vi "client.vi"() -> ()   [LabVIEW 2019]
uses:
  Generated_client/RPC Messages/Greeter_req.ctl
  Generated_client/RPC Messages/Greeter_req_req_oneof/Greeter_req_req_oneof.lvclass
  Generated_client/RPC Messages/Greeter_req_req_oneof/Greeter_req_req_oneof.lvclass/Greeter_req_req_oneof.ctl
  Generated_client/RPC Messages/Greeter_MessageA.ctl
  Generated_client/RPC Messages/Greeter_MessageA_oneof_a/Greeter_MessageA_oneof_a.lvclass
  Generated_client/RPC Messages/Greeter_MessageA_oneof_a/Greeter_MessageA_oneof_a.lvclass/Greeter_MessageA_oneof_a.ctl
  Generated_client/RPC Messages/Greeter_res_res_oneof/Greeter_res_res_oneof.lvclass/Greeter_res_res_oneof.ctl
  Generated_client/Generated_client.lvlib
  Generated_client/RPC Messages/Greeter_res_res_oneof/Greeter_res_res_oneof.lvclass
panel:
  in  "oneof_a":i32(ring)=2 items=["data_a1"=1, "data_a2"=2]
  in  "req_omeof":i32(ring)=2 items=["req_price"=3, "message_a"=2]
  out "res_price":dbl format="%.2f"
  out "res_data_a2":string
  out "res_data_a1":string
  out "res_anotherField":string
  out "res_id":i32
  in  "error in":errorcluster
  out "error out":errorcluster
  in  "data_a2":string="abc"
  in  "data_a1":string="bca"
  in  "anotherField":string="hi"
  in  "req_price":dbl=101.1
  in  "req_id":i32=101
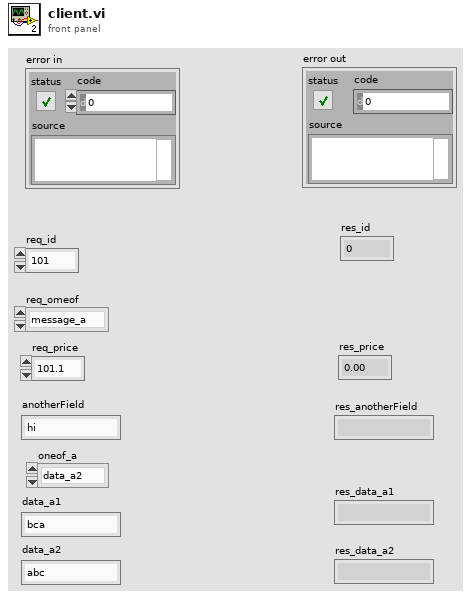
[diagram p1: front panel]
types:
  T1 = typedef "Generated_client.lvlib/Greeter_req.ctl" = cluster{"req_id":i32, "Greeter_req_req_oneof":refnum<class "Greeter_req_req_oneof.lvclass">}
  T2 = typedef "Generated_client.lvlib/Greeter_MessageA.ctl" = cluster{"anotherField":string, "Greeter_MessageA_oneof_a":refnum<class "Greeter_MessageA_oneof_a.lvclass">}
  T3 = typedef "grpc-lvsupport-release.lvlib/grpcId.ctl" = u64
  T4 = typedef "Generated_client.lvlib/Greeter_res.ctl" = cluster{"res_id":i32, "Greeter_res_res_oneof":refnum<class "Greeter_res_res_oneof.lvclass">}
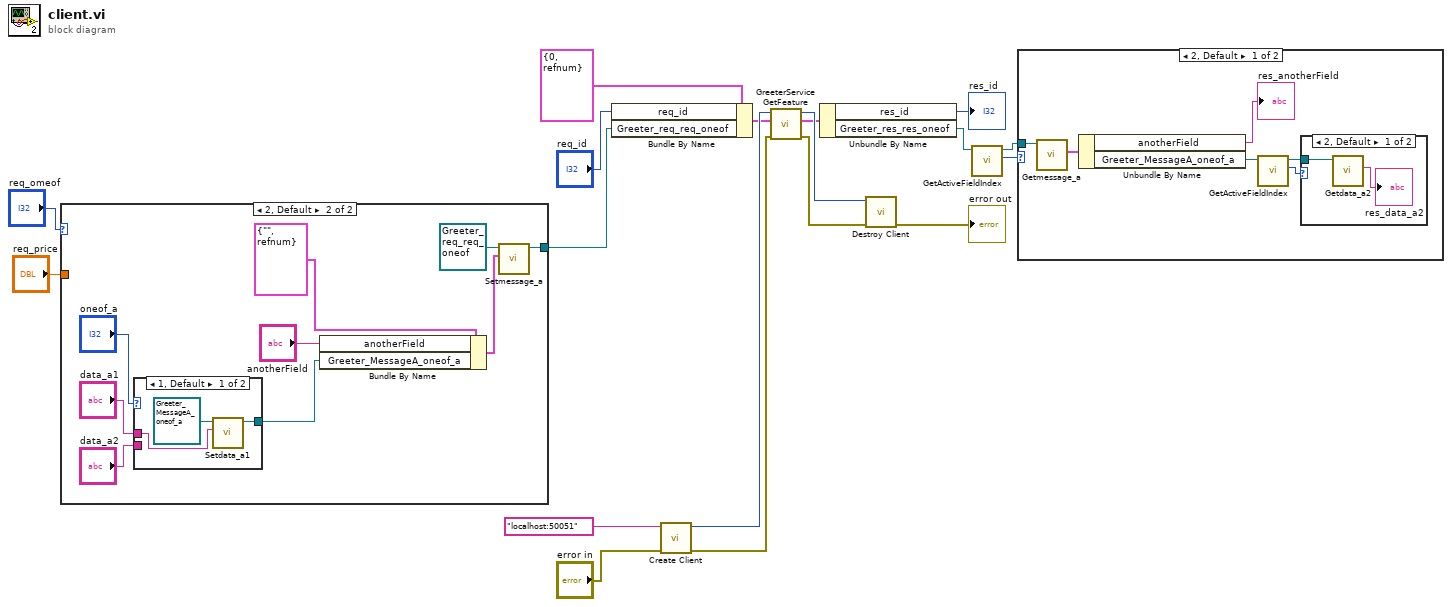
[diagram p0: block diagram]
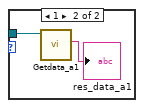
[diagram p2: hidden frame]
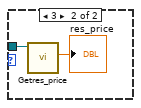
[diagram p3: hidden frame]
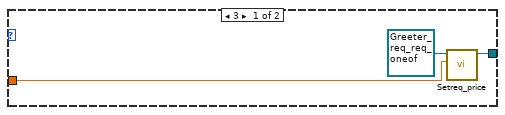
[diagram p4: hidden frame]
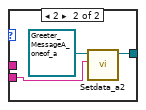
[diagram p5: hidden frame]
diagram:
  n1 = case shown="2, Default" "req_omeof" {
    tunnel: "req_price" -> [w21 _]
    tunnel: [w19 w23] -> w10
    frame 3 {
      n2 = call "Setreq_price.vi"("Set_Val"=w21, "OneOfTemplate in"=refnum<class "Greeter_req_req_oneof.lvclass"> refnum) -> ("OneOfTemplate out"=w19:refnum<class "Greeter_req_req_oneof.lvclass">)  [unwired: 8 in, 1 out]
    }
    frame 2, Default {
      n3 = case shown="1, Default" "oneof_a" {
        tunnel: "data_a1" -> [w33 _]
        tunnel: [w31 w34] -> w26
        tunnel: "data_a2" -> [_ w36]
        frame 1, Default {
          n4 = call "Setdata_a1.vi"("Set_Val"=w33, "OneOfTemplate in"=refnum<class "Greeter_MessageA_oneof_a.lvclass"> refnum) -> ("OneOfTemplate out"=w31:refnum<class "Greeter_MessageA_oneof_a.lvclass">)  [unwired: 8 in, 1 out]
        }
        frame 2 {
          n5 = call "Setdata_a2.vi"("Set_Val"=w36, "OneOfTemplate in"=refnum<class "Greeter_MessageA_oneof_a.lvclass"> refnum) -> ("OneOfTemplate out"=w34:refnum<class "Greeter_MessageA_oneof_a.lvclass">)  [unwired: 8 in, 1 out]
        }
      }
      n6 = Bundle By Name(cluster=T2 {"anotherField"="", "Greeter_MessageA_oneof_a"=refnum} ("Greeter_MessageA"), "anotherField"="anotherField", "Greeter_MessageA_oneof_a"=w26) -> (w25:T2)
      n7 = call "Setmessage_a.vi"("Set_Val"=w25, "OneOfTemplate in"=refnum<class "Greeter_req_req_oneof.lvclass"> refnum) -> ("OneOfTemplate out"=w23:refnum<class "Greeter_req_req_oneof.lvclass">)  [unwired: 8 in, 1 out]
    }
  }
  n8 = Bundle By Name(cluster=T1 {"req_id"=0, "Greeter_req_req_oneof"=refnum} ("Greeter_req"), "req_id"="req_id", "Greeter_req_req_oneof"=w10) -> (w7:T1)
  n9 = call "Create Client.vi"("error in"="error in", "address"="localhost:50051") -> ("error out"=w18:errorcluster, "gRPC ID Out"=w13:T3)  [unwired: 8 in]
  n10 = call "GreeterService GetFeature.vi"("error in"=w18, "Request Data"=w7, "gRPC ID"=w13) -> ("error out"=w17:errorcluster, "Response Data"=w6:T4, "gRPC ID out"=w12:T3)  [unwired: 6 in]
  n11 = Unbundle By Name(w6) -> ("res_id"=→"res_id":i32, "Greeter_res_res_oneof"=w4:refnum<class "Greeter_res_res_oneof.lvclass">)
  n12 = call "Destroy Client.vi"("error in"=w17, "gRPC ID"=w12) -> ("error out"=→"error out":errorcluster)  [unwired: 9 in]
  n13 = call "GetActiveFieldIndex.vi"("OneOfTemplate in"=w4) -> ("Active Field Index"=w2:i32, "OneOfTemplate out"=w3:refnum<class "Greeter_res_res_oneof.lvclass">)  [unwired: 8 in, 1 out]
  n14 = case shown="2, Default" w2 {
    tunnel: w3 -> [w38 w48]
    frame 2, Default {
      n15 = call "Getmessage_a.vi"("OneOfTemplate in"=w38) -> ("Get_Val"=w42:T2)  [unwired: 8 in, 2 out]
      n16 = Unbundle By Name(w42) -> ("anotherField"=→"res_anotherField":string, "Greeter_MessageA_oneof_a"=w40:refnum<class "Greeter_MessageA_oneof_a.lvclass">)
      n17 = call "GetActiveFieldIndex.vi"("OneOfTemplate in"=w40) -> ("Active Field Index"=w39:i32, "OneOfTemplate out"=w37:refnum<class "Greeter_MessageA_oneof_a.lvclass">)  [unwired: 8 in, 1 out]
      n18 = case shown="2, Default" w39 {
        tunnel: w37 -> [w44 w46]
        frame 2, Default {
          n19 = call "Getdata_a2.vi"("OneOfTemplate in"=w44) -> ("Get_Val"=→"res_data_a2":string)  [unwired: 8 in, 2 out]
        }
        frame 1 {
          n20 = call "Getdata_a1.vi"("OneOfTemplate in"=w46) -> ("Get_Val"=→"res_data_a1":string)  [unwired: 8 in, 2 out]
        }
      }
    }
    frame 3 {
      n21 = call "Getres_price.vi"("OneOfTemplate in"=w48) -> ("Get_Val"=→"res_price":dbl)  [unwired: 8 in, 2 out]
    }
  }
